vi "Package Information Pre Build Action.vi"(10 "Variant":variant) -> (0 "error out":errorcluster)   [LabVIEW 2017, in "CL_G3_VIComponentBuilder.lvlib"]
uses:
  CL_G3_VIComponentBuilder.lvlib
  <vilib>/LVH/i3 JSON/JSON Parsing/Get Object Parameter Files/Get Object Parameter - Object.vi
  <vilib>/LVH/i3 JSON/JSON Parsing/Get Object Parameter Files/Get Object Parameter - Boolean.vi
  VIPM Utilities/CL_G3_VIPMUtilities.lvlib
  <vilib>/LVH/i3 JSON/i3-json.lvlib
panel:
  out "String":string
  out "Total":i32
  out "Progress":i32(slide) scale=-1.0..85.0
  # "Adding Package details to VI description"
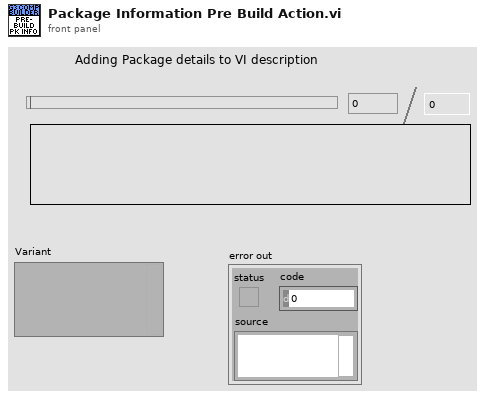
[diagram p1: front panel]
types:
  T1 = enum32{"Invalid", "Standard", "Closed", "Hidden", "Minimized", "Maximized"}
  T2 = cluster{"Error State":errorcluster, "Processed Documentation":string, "Build Spec Path":path, "VIs In Package":path[], "Product Name":string, "Package Version":string, "Package Name":string, "Current File to process":path, "vi reference being processed":refnum<vi>, "Opened References":refnum<vi>[], "Build Options i3JSON Tree":variant}
  T3 = cluster{"Beginning of Tag Position":i32, "End of Tag Position":i32}[]
  T4 = cluster{"Beginning of Tag Position":i32, "End of Tag Position":i32}
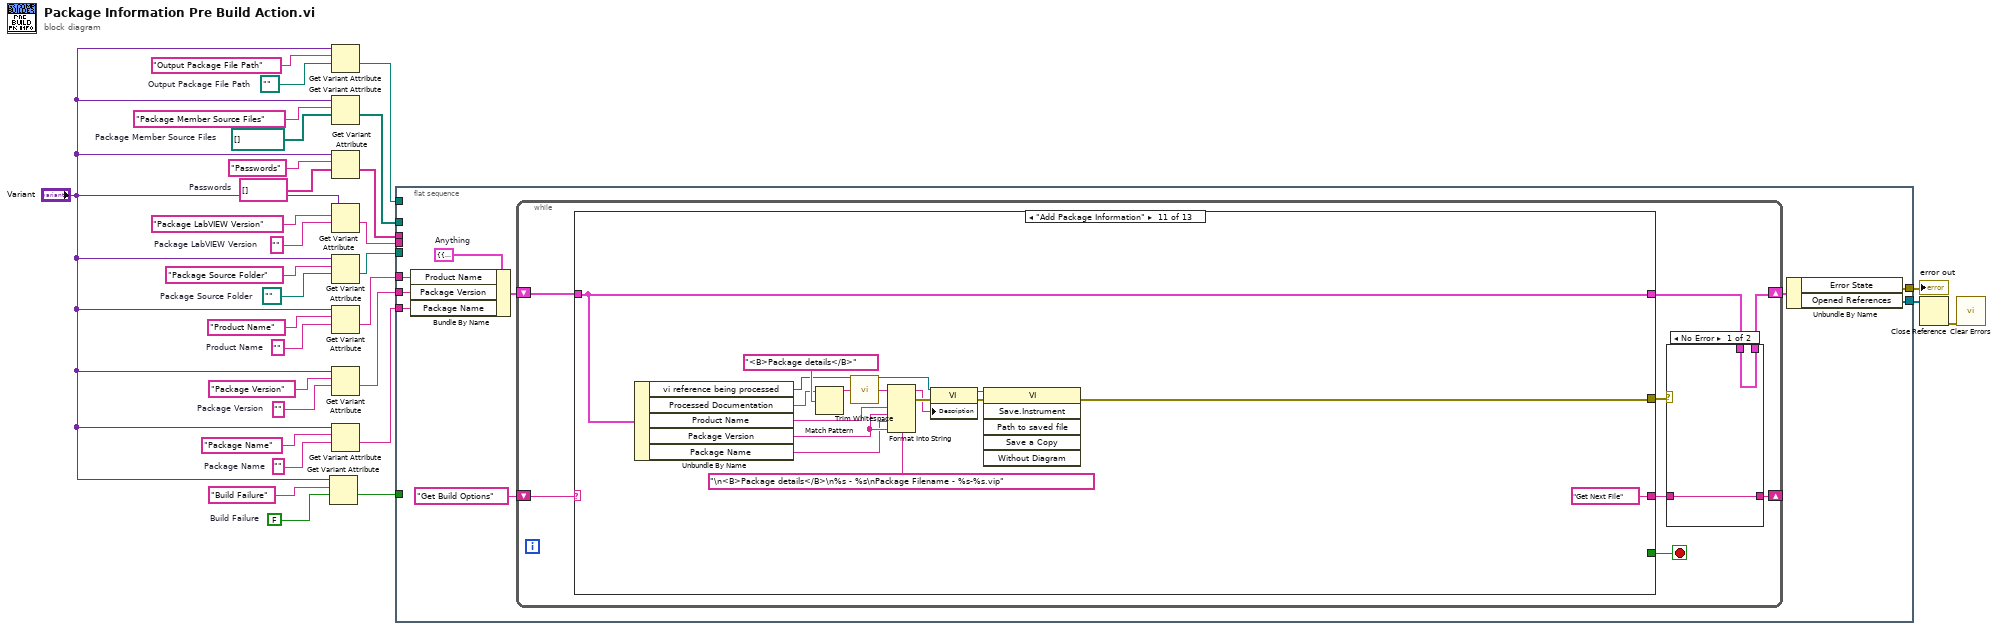
[diagram p0: block diagram]
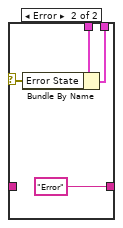
[diagram p2: hidden frame]
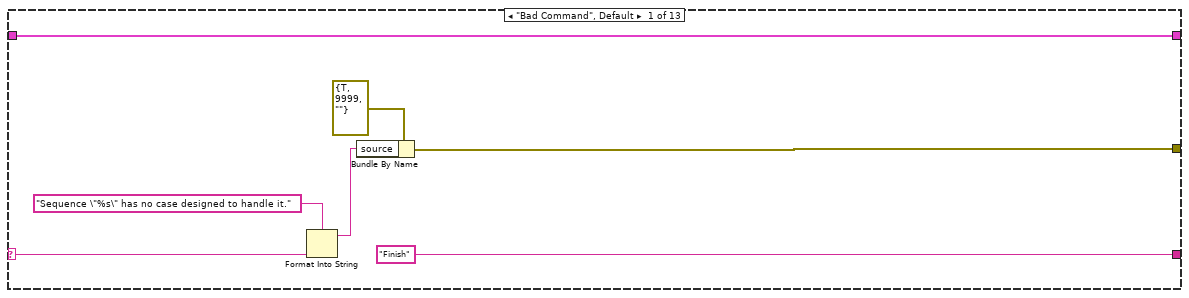
[diagram p3: hidden frame]
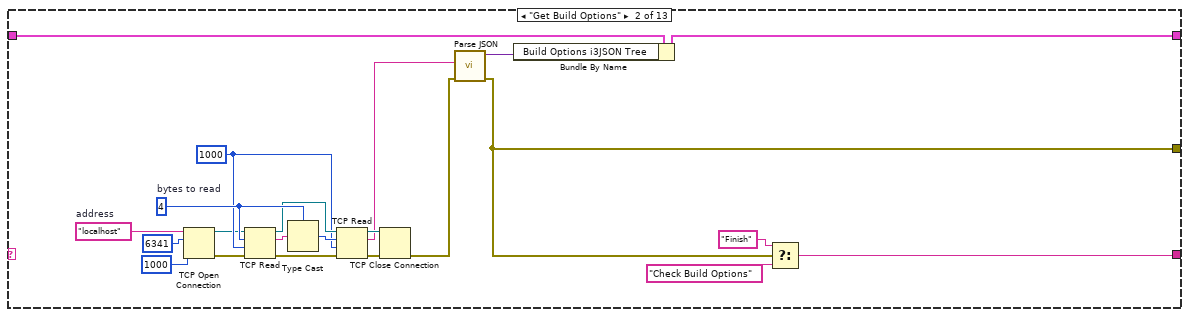
[diagram p4: hidden frame]
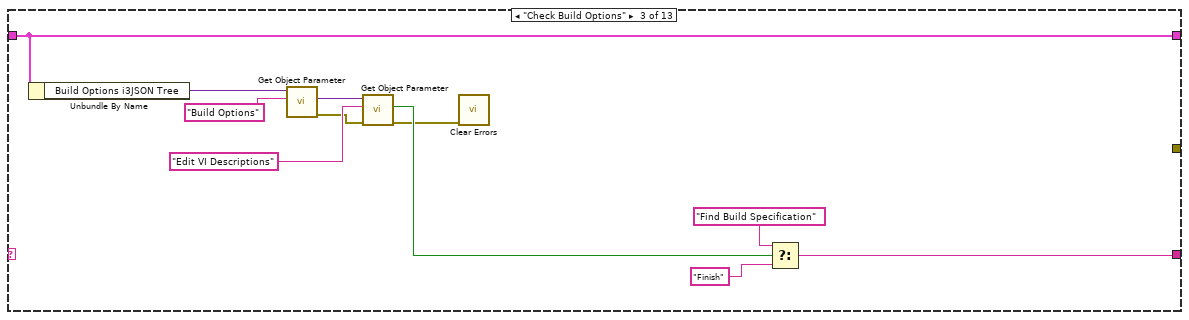
[diagram p5: hidden frame]
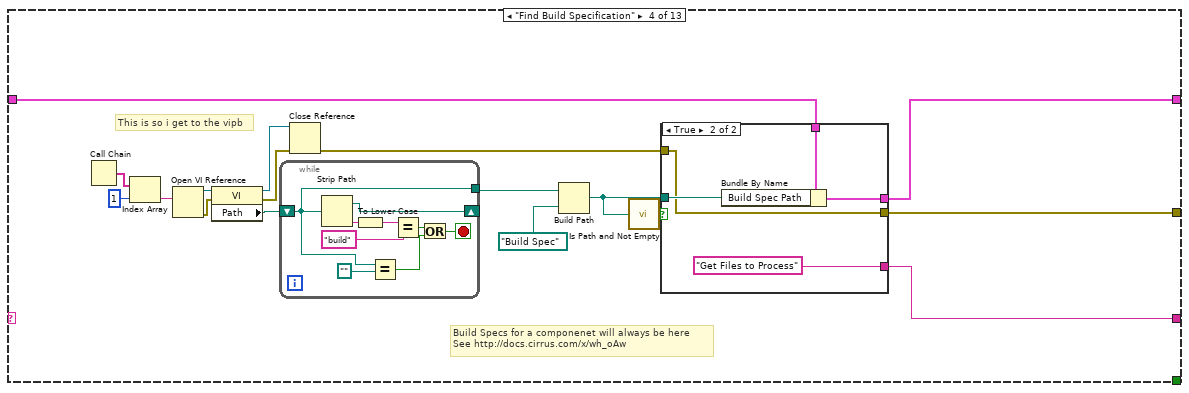
[diagram p6: hidden frame]
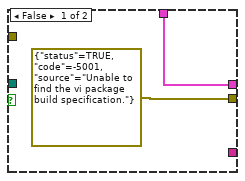
[diagram p7: hidden frame]
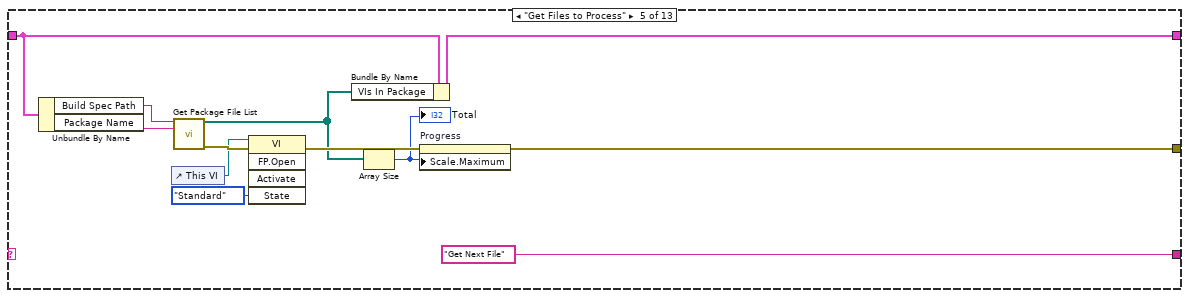
[diagram p8: hidden frame]
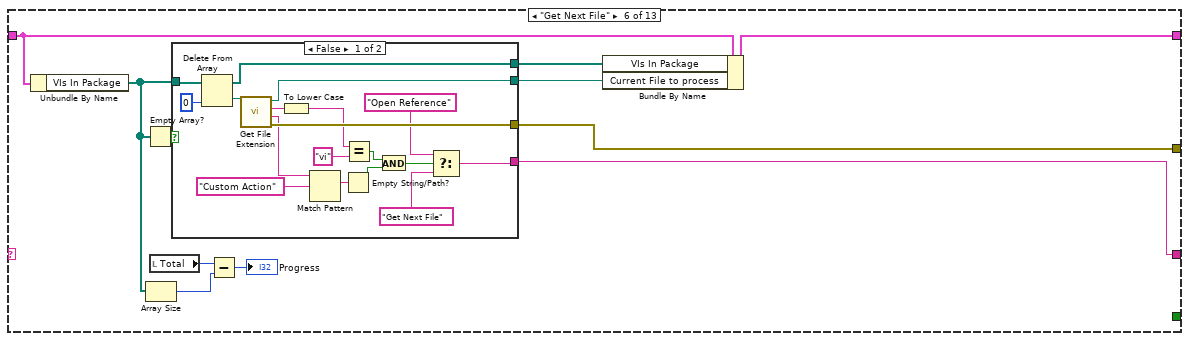
[diagram p9: hidden frame]
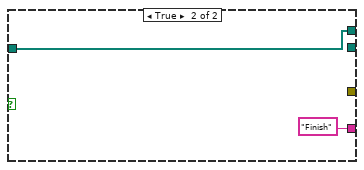
[diagram p10: hidden frame]
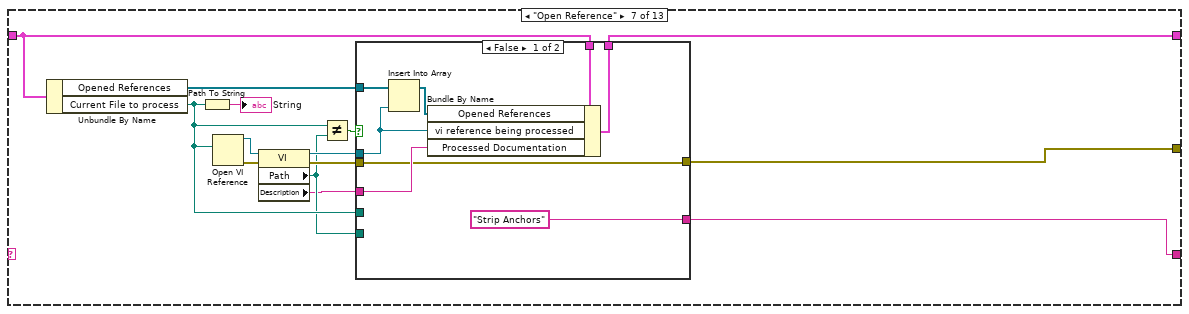
[diagram p11: hidden frame]
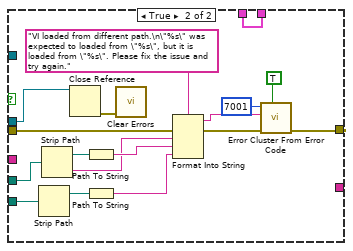
[diagram p12: hidden frame]
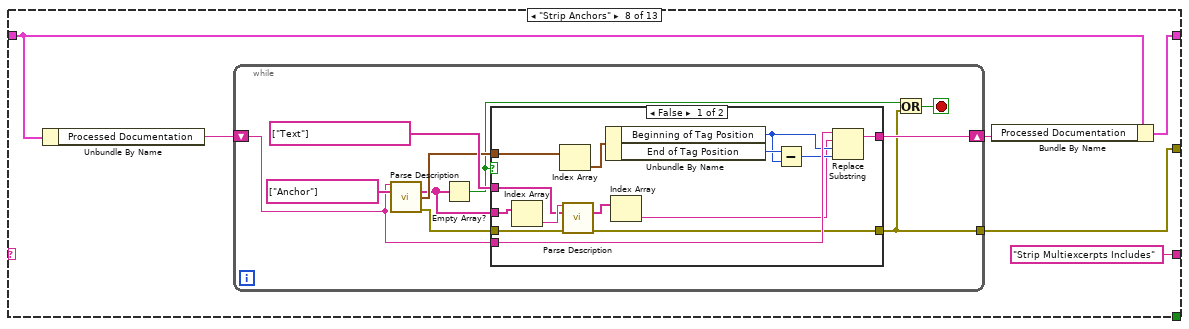
[diagram p13: hidden frame]
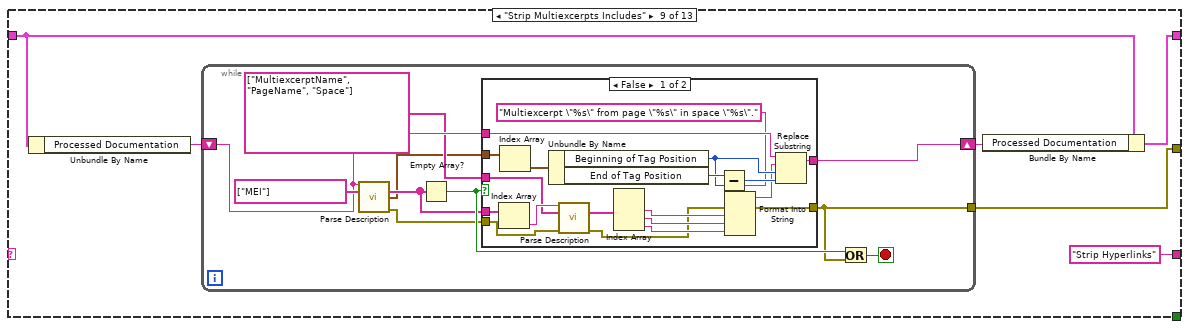
[diagram p15: hidden frame]
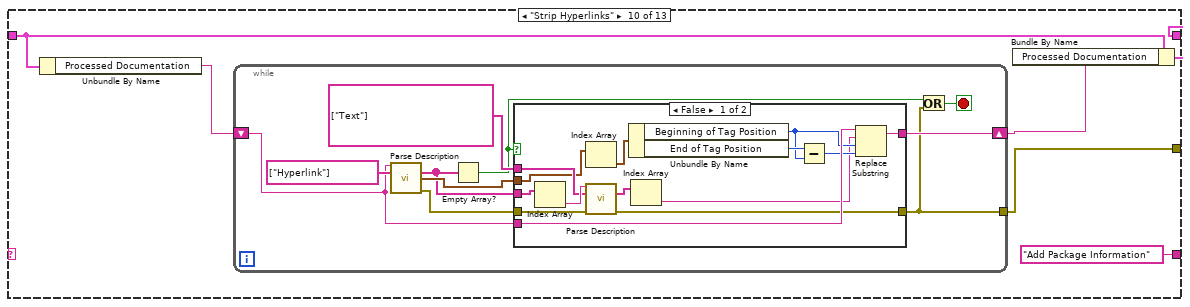
[diagram p17: hidden frame]
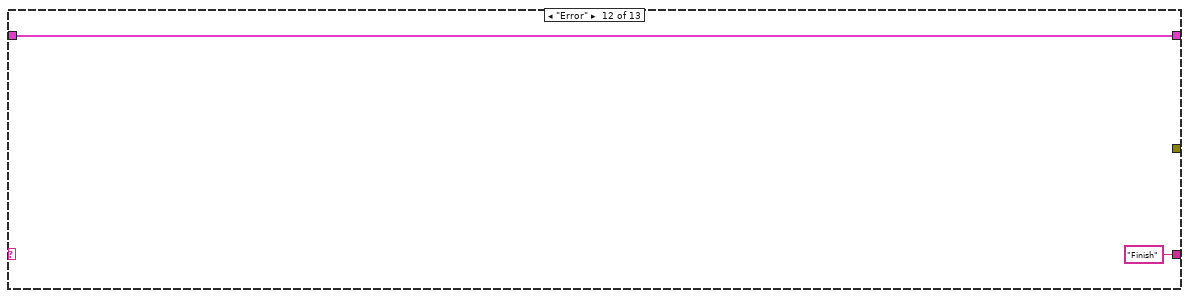
[diagram p19: hidden frame]
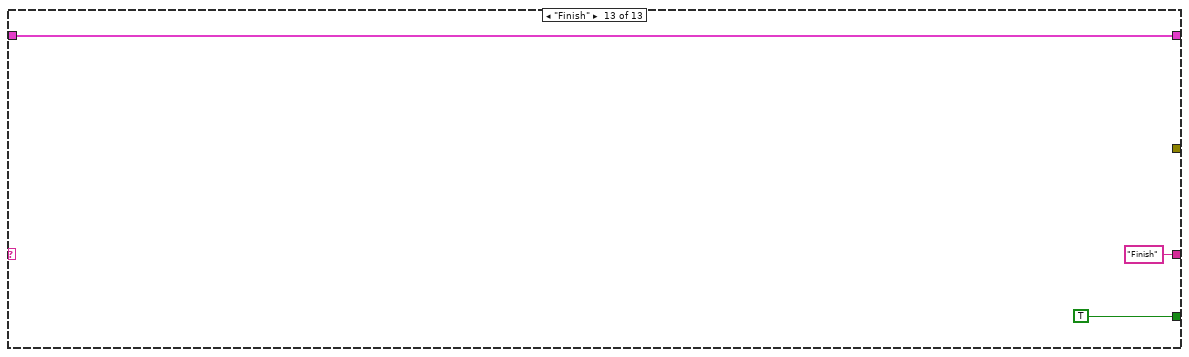
[diagram p20: hidden frame]
diagram:
  w14 = FALSE  # Build Failure
  w16 = path ""  # Package Source Folder
  w17 = ""  # Package Name
  w20 = ""  # Package LabVIEW Version
  w22 = ""  # Package Version
  w24 = ""  # Product Name
  w26 = string[] []  # Passwords
  w28 = path[] []  # Package Member Source Files
  w30 = path ""  # Output Package File Path
  n1 = Get Variant Attribute(Variant="Variant", name="Build Failure", default value (empty Variant)=w14) -> (value=w1:bool)  [unwired: 1 in, 3 out]
  n2 = Get Variant Attribute(Variant="Variant", name="Output Package File Path", default value (empty Variant)=w30) -> (value=w6:path)  [unwired: 1 in, 3 out]
  n3 = Get Variant Attribute(Variant="Variant", name="Package Member Source Files", default value (empty Variant)=w28) -> (value=w5:path[])  [unwired: 1 in, 3 out]
  n4 = Get Variant Attribute(Variant="Variant", name="Passwords", default value (empty Variant)=w26) -> (value=w4:string[])  [unwired: 1 in, 3 out]
  n5 = Get Variant Attribute(Variant="Variant", name="Package LabVIEW Version", default value (empty Variant)=w20) -> (value=w3:string)  [unwired: 1 in, 3 out]
  n6 = Get Variant Attribute(Variant="Variant", name="Package Source Folder", default value (empty Variant)=w16) -> (value=w2:path)  [unwired: 1 in, 3 out]
  n7 = Get Variant Attribute(Variant="Variant", name="Product Name", default value (empty Variant)=w24) -> (value=w12:string)  [unwired: 1 in, 3 out]
  n8 = Get Variant Attribute(Variant="Variant", name="Package Version", default value (empty Variant)=w22) -> (value=w11:string)  [unwired: 1 in, 3 out]
  n9 = Get Variant Attribute(Variant="Variant", name="Package Name", default value (empty Variant)=w17) -> (value=w10:string)  [unwired: 1 in, 3 out]
  n10 = flat-sequence {
    tunnel: w12 -> [w38]
    tunnel: w11 -> [w37]
    tunnel: w10 -> [w36]
    tunnel: [w34] -> w9
    tunnel: [w33] -> w8
    tunnel: w6 -> [_]
    tunnel: w5 -> [_]
    tunnel: w4 -> [_]
    tunnel: w3 -> [_]
    tunnel: w2 -> [_]
    tunnel: w1 -> [_]
    frame #0 {
      w32 = T2 {"Error State"={"status"=FALSE, "code"=0, "source"=""}, "Processed Documentation"="", "Build Spec Path"=path "", "VIs In Package"=[], "Product Name"="", "Package Version"="", "Package Name"="", "Current File to process"=path "", "vi reference being processed"=refnum, "Opened References"=[], "Build Options i3JSON Tree"=variant}  # Anything
      n11 = Bundle By Name(cluster=w32, "Product Name"=w38, "Package Version"=w37, "Package Name"=w36) -> (w40:T2)
      n12 = while {
        shift-right: [w43] -> w39
        shift-left: w40 -> [w48]
        shift-right: [w42] -> _
        shift-left: "Get Build Options" -> [w47]
        stop <- w41 stop-if-true
        n13 = case shown="\"Add Package Information\"" w47 {
          selector: w47 -> [w58 _ _ _ _ _ _ _ _ _ _ _ _]
          tunnel: w48 -> [w61 w83 w91 w100 w131 w150 w175 w215 w246 w283 w315 w326 w329]
          tunnel: [w61 w67 w91 w101 w135 w149 w174 w213 w244 w281 w315 w326 w329] -> w44
          tunnel: ["Finish" ("Accessors:Name") w82 w92 w99 "Get Next File" w145 w173 "Strip Multiexcerpts Includes" ("y") "Strip Hyperlinks" ("y") "Add Package Information" ("y") "Get Next File" ("y") "Finish" "Finish"] -> w46
          tunnel: [w56 w64 _ w97 w133 w147 w178 w211 w241 w278 w310 _ _] -> w45
          tunnel: [_ _ _ _ _ _ _ _ _ _ _ _ TRUE] -> w41
          frame "Bad Command", Default {
            n14 = Format Into String(format string="Sequence \"%s\" has no case designed to handle it.", w58) -> (resulting string=w57:string)  [unwired: 2 in, 1 out]
            n15 = Bundle By Name(cluster=errorcluster {"status"=TRUE, "code"=9999, "source"=""} ("error out"), "source"=w57) -> (w56:errorcluster)
          }
          frame "Get Build Options" {
            w74 = 1000 ("timeout ms (25000)")
            w78 = 4  # bytes to read
            w81 = "localhost"  # address
            n16 = TCP Open Connection(address=w81, remote port or service name=u16 6341, timeout ms (60000)=1000) -> (connection ID=w73:refnum<k5>, error out=w72:errorcluster)  [unwired: 2 in]
            n17 = TCP Read(connection ID=w73, bytes to read=w78, error in (no error)=w72, 9:w74) -> (connection ID out=w77:refnum<k5>, data out=w79:string, error out=w76:errorcluster)  [unwired: 1 in]
            n18 = Type Cast(type=w78, x=w79) -> (*(type *) &x=w75:i32)
            n19 = TCP Read(connection ID=w77, bytes to read=w75, error in (no error)=w76, 9:w74) -> (connection ID out=w71:refnum<k5>, data out=w69:string, error out=w70:errorcluster)  [unwired: 1 in]
            n20 = TCP Close Connection(connection ID=w71, error in (no error)=w70) -> (error out=w65:errorcluster)  [unwired: 1 in, 1 out]
            n21 = call <vilib>:"Parse JSON.vi"("error in (no error)"=w65, "JSON String"=w69) -> ("error out"=w64:errorcluster, "JSON Tree"=w66:variant)  [unwired: 6 in, 2 out]
            n22 = Bundle By Name(cluster=w83, "Build Options i3JSON Tree"=w66) -> (w67:T2)
            n23 = Select(t="Finish", s=w64, f="Check Build Options") -> (s? t:f=w82:string)
          }
          frame "Check Build Options" {
            n24 = Unbundle By Name(w91) -> ("Build Options i3JSON Tree"=w90:variant)
            n25 = call-poly <vilib>:"Get Object Parameter.vi"("Parameter Name"="Build Options", "JSON Tree In (JSON Object)"=w90) -> ("error out"=w85:errorcluster, "JSON Object"=w89:variant)  [unwired: 6 in, 2 out]
            n26 = call-poly <vilib>:"Get Object Parameter.vi"("error in (no error)"=w85, "Parameter Name"="Edit VI Descriptions" ("Option Name"), "JSON Tree In (JSON Object)"=w89) -> ("error out"=w84:errorcluster, "Boolean Value"=w86:bool)  [unwired: 5 in, 2 out]
            n27 = call <vilib>:"Clear Errors.vi"("error in (no error)"=w84) -> ()  [unwired: 5 in, 2 out]
            n28 = Select(t="Find Build Specification", s=w86, f="Finish") -> (s? t:f=w92:string)
          }
          frame "Find Build Specification" {
            # "This is so i get to the vipb"
            # "Build Specs for a componenet will always be here\nSee http://docs.cirrus.com/x/wh_oAw"
            n29 = Call Chain() -> (call chain=w109:string[])
            n30 = Index Array(array=w109, index=1) -> (element=w105:string)
            n31 = Open VI Reference(vi path=w105) -> (vi reference=w106:refnum<vi>, error out=w98:errorcluster)  [unwired: 5 in]
            n32 = property class="VI"(reference=w106, error in=w98) -> (reference out=w107:refnum<vi>, error out=w96:errorcluster, "Path"=w108:path)
            n33 = while {
              shift-right: [w122] -> _
              shift-left: w108 -> [w120]
              tunnel: [w120] -> w111
              stop <- w127 stop-if-true
              n34 = Strip Path(path=w120) -> (stripped path=w122:path, name=w126:string)
              n35 = To Lower Case(string=w126) -> (all lower case string=w125:string)
              n36 = Equal?(x=w120, y=path "") -> (x = y?=w119:bool)
              n37 = Equal?(x=w125, y="build") -> (x = y?=w123:bool)
              n38 = Or(x=w123, y=w119) -> (x .or. y?=w127:bool)
            }
            n39 = Close Reference(reference=w107, error in (no error)=w96) -> (error out=w95:errorcluster)
            n40 = Build Path(base path=w111, name or relative path=path "Build Spec" ("VIPB Folder")) -> (appended path=w102:path)
            n41 = call <vilib>:"Is Path and Not Empty.vi"("path"=w102) -> ("Is Path and Not Empty?"=w103:bool)  [unwired: 4 in]
            n42 = case shown="True" w103 {
              tunnel: [_ "Get Files to Process"] -> w99
              tunnel: w102 -> [_ w117]
              tunnel: w100 -> [w112 w116]
              tunnel: [w112 w115] -> w101
              tunnel: [errorcluster {"status"=TRUE, "code"=-5001, "source"="Unable to find the vi package build specification."} ("Error State") w114] -> w97
              tunnel: w95 -> [_ w114]
              frame False {
              }
              frame True {
                n43 = Bundle By Name(cluster=w116, "Build Spec Path"=w117) -> (w115:T2)
              }
            }
          }
          frame "Get Files to Process" {
            n44 = Unbundle By Name(w131) -> ("Build Spec Path"=w130:path, "Package Name"=w129:string)
            n45 = control-ref of="This VI"() -> (w136:refnum<vi>)
            n46 = call "Get Package File List.vi"("VIPB Folder"=w130, "Package Name"=w129) -> ("Included Files"=w134:path[], "error out"=w139:errorcluster)  [unwired: 12 in]
            n47 = invoke class="VI" method="FP.Open"(reference=w136, error in=w139, "State"=T1."Standard") -> (error out=w138:errorcluster)  [unwired: 2 in, 4 out]
            n48 = Bundle By Name(cluster=w131, "VIs In Package"=w134) -> (w135:T2)
            n49 = Array Size(array=w134) -> (size(s)=w132:i32)
            "Total" <- w132
            n50 = property on="Progress" class="Slide (strict)"(error in=w138, "Scale.Maximum"=w132) -> (error out=w133:errorcluster)  [unwired: 1 in, 1 out]
          }
          frame "Get Next File" {
            n51 = Unbundle By Name(w150) -> ("VIs In Package"=w143:path[])
            n52 = Empty Array?(array=w143) -> (empty?=w146:bool)
            n53 = Array Size(array=w143) -> (size(s)=w142:i32)
            n54 = local read "Total"() -> (w141:i32)
            n55 = case shown="False" w146 {
              tunnel: [w165 _] -> w148
              tunnel: [w164 _] -> w147
              tunnel: w143 -> [w157 w169]
              tunnel: [w153 "Finish" ("y")] -> w145
              tunnel: [w152 w169] -> w144
              frame False {
                n56 = Delete From Array(array=w157, index=0) -> (deleted portion=w166:path, array with subset deleted=w152:path[])  [unwired: 1 in]
                n57 = call <vilib>:"Get File Extension.vi"("file"=w166) -> ("error out"=w164:errorcluster, "filename without extension"=w163:string, "lowercase file extension"=w162:string, "dup file"=w165:path)  [unwired: 6 in, 1 out]
                n58 = To Lower Case(string=w162) -> (all lower case string=w160:string)
                n59 = Match Pattern(string=w163, regular expression="Custom Action") -> (match substring=w168:string)  [unwired: 1 in, 3 out]
                n60 = Empty String/Path?(string/path=w168) -> (empty?=w158:bool)
                n61 = Equal?(x=w160, y="vi") -> (x = y?=w159:bool)
                n62 = And(x=w159, y=w158) -> (x .and. y?=w156:bool)
                n63 = Select(t="Open Reference" ("y"), s=w156, f="Get Next File" ("y")) -> (s? t:f=w153:string)
              }
              frame True {
              }
            }
            n64 = Subtract(x=w141, y=w142) -> (x-y=→"Progress":i32)
            n65 = Bundle By Name(cluster=w150, "VIs In Package"=w144, "Current File to process"=w148) -> (w149:T2)
          }
          frame "Open Reference" {
            n66 = Unbundle By Name(w175) -> ("Opened References"=w171:refnum<vi>[], "Current File to process"=w177:path)
            n67 = Path To String(path=w177) -> (string=→"String":string)
            n68 = Open VI Reference(vi path=w177) -> (vi reference=w184:refnum<vi>, error out=w183:errorcluster)  [unwired: 5 in]
            n69 = property class="VI"(reference=w184, error in=w183) -> (reference out=w180:refnum<vi>, error out=w179:errorcluster, "Path"=w176:path, "Description"=w172:string)
            n70 = Not Equal?(x=w177, y=w176) -> (x != y?=w181:bool)
            n71 = case shown="False" w181 {
              tunnel: w180 -> [w187 w195]
              tunnel: w179 -> [w185 w199]
              tunnel: [w185 w198] -> w178
              tunnel: w177 -> [_ w197]
              tunnel: w176 -> [_ w196]
              tunnel: w175 -> [w192 w193]
              tunnel: [w191 w193] -> w174
              tunnel: ["Strip Anchors" _] -> w173
              tunnel: w172 -> [w189 _]
              tunnel: w171 -> [w188 _]
              frame False {
                n72 = Insert Into Array(array=w188, new element=w187) -> (w186:refnum<vi>[])  [unwired: 1 in]
                n73 = Bundle By Name(cluster=w192, "Opened References"=w186, "vi reference being processed"=w187, "Processed Documentation"=w189) -> (w191:T2)
              }
              frame True {
                n74 = Strip Path(path=w196) -> (stripped path=w205:path)  [unwired: 1 out]
                n75 = Strip Path(path=w197) -> (stripped path=w203:path, name=w202:string)
                n76 = Close Reference(reference=w195) -> (error out=w194:errorcluster)  [unwired: 1 in]
                n77 = Path To String(path=w203) -> (string=w204:string)
                n78 = Path To String(path=w205) -> (string=w206:string)
                n79 = call <vilib>:"Clear Errors.vi"("error in (no error)"=w194) -> ()  [unwired: 5 in, 2 out]
                n80 = Format Into String(format string="VI loaded from different path.\n\"%s\" was expected to loaded from \"%s\", but it is loaded from \"%s\". Please fix the issue and try again.", error in=w199, w202, w204, w206) -> (resulting string=w207:string, error out=w200:errorcluster)  [unwired: 1 in]
                n81 = call <vilib>:"Error Cluster From Error Code.vi"("show call chain? (False)"=TRUE, "error in (no error)"=w200, "error message (\"\")"=w207, "error code (0)"=7001) -> ("error out"=w198:errorcluster)  [unwired: 5 in]
              }
            }
          }
          frame "Strip Anchors" {
            n82 = Unbundle By Name(w215) -> ("Processed Documentation"=w214:string)
            n83 = while {
              shift-right: [w221] -> w212
              shift-left: w214 -> [w222]
              tunnel: [w218] -> w211
              stop <- w216 stop-if-true
              n84 = call "Parse Description.vi"("Description"=w222, "XML Values to Parse"=string[] ["Anchor"]) -> ("XML Values"=w219:string[], "String Bounds of Matches"=w223:T3, "error out"=w220:errorcluster)  [unwired: 10 in, 1 out]
              n85 = Empty Array?(array=w219) -> (empty?=w217:bool)
              n86 = case shown="False" w217 {
                tunnel: w219 -> [w239 _]
                tunnel: w220 -> [w236 _]
                tunnel: string[] ["Text"] ("XML Values to Parse") -> [w235 _]
                tunnel: w223 -> [w234 _]
                tunnel: w222 -> [w233 w240]
                tunnel: [w232 w240] -> w221
                tunnel: [w226 _] -> w218
                frame False {
                  n87 = Index Array(array=w239) -> (element=w238:string)  [unwired: 1 in]
                  n88 = Index Array(array=w234) -> (element=w231:T4)  [unwired: 1 in]
                  n89 = call "Parse Description.vi"("Description"=w238, "XML Values to Parse"=w235, "error in (no error) 2"=w236) -> ("XML Values"=w237:string[], "error out"=w226:errorcluster)  [unwired: 9 in, 2 out]
                  n90 = Unbundle By Name(w231) -> ("Beginning of Tag Position"=w229:i32, "End of Tag Position"=w230:i32)
                  n91 = Index Array(array=w237) -> (element=w227:string)  [unwired: 1 in]
                  n92 = Subtract(x=w230, y=w229) -> (x-y=w228:i32)
                  n93 = Replace Substring(2:w228, 3:w229, 4:w227, 5:w233) -> (1:w232:string)  [unwired: 1 out]
                }
                frame True {
                }
              }
              n94 = Or(x=w217, y=w218) -> (x .or. y?=w216:bool)
            }
            n95 = Bundle By Name(cluster=w215, "Processed Documentation"=w212) -> (w213:T2)
          }
          frame "Strip Multiexcerpts Includes" {
            n96 = Unbundle By Name(w246) -> ("Processed Documentation"=w245:string)
            n97 = while {
              shift-right: [w254] -> w243
              shift-left: w245 -> [w255]
              tunnel: [w247] -> w241
              stop <- w252 stop-if-true
              n98 = call "Parse Description.vi"("Description"=w255, "XML Values to Parse"=string[] ["MEI"]) -> ("XML Values"=w251:string[], "String Bounds of Matches"=w249:T3, "error out"=w248:errorcluster)  [unwired: 10 in, 1 out]
              n99 = Empty Array?(array=w251) -> (empty?=w253:bool)
              n100 = case shown="False" w253 {
                tunnel: w249 -> [w275 _]
                tunnel: w255 -> [w274 w277]
                tunnel: [w273 w277] -> w254
                tunnel: w251 -> [w268 _]
                tunnel: string[] ["MultiexcerptName", "PageName", "Space"] ("XML Values to Parse") -> [w266 _]
                tunnel: [w258 w276] -> w247
                tunnel: w248 -> [w257 w276]
                frame False {
                  n101 = Index Array(array=w268) -> (element=w267:string)  [unwired: 1 in]
                  n102 = Index Array(array=w275) -> (element=w272:T4)  [unwired: 1 in]
                  n103 = Unbundle By Name(w272) -> ("Beginning of Tag Position"=w270:i32, "End of Tag Position"=w271:i32)
                  n104 = call "Parse Description.vi"("Description"=w267, "XML Values to Parse"=w266, "error in (no error) 2"=w257) -> ("XML Values"=w265:string[], "error out"=w259:errorcluster)  [unwired: 9 in, 2 out]
                  n105 = Index Array(array=w265) -> (element #1=w264:string, element #2=w263:string, element #3=w262:string)  [unwired: 3 in]
                  n106 = Subtract(x=w271, y=w270) -> (x-y=w269:i32)
                  n107 = Format Into String(format string="Multiexcerpt \"%s\" from page \"%s\" in space \"%s\".", error in=w259, w264, w263, w262) -> (resulting string=w260:string, error out=w258:errorcluster)  [unwired: 1 in]
                  n108 = Replace Substring(2:w269, 3:w270, 4:w260, 5:w274) -> (1:w273:string)  [unwired: 1 out]
                }
                frame True {
                }
              }
              n109 = Or(x=w253, y=w247) -> (x .or. y?=w252:bool)
            }
            n110 = Bundle By Name(cluster=w246, "Processed Documentation"=w243) -> (w244:T2)
          }
          frame "Strip Hyperlinks" {
            n111 = Unbundle By Name(w283) -> ("Processed Documentation"=w282:string)
            n112 = while {
              shift-right: [w289] -> w280
              shift-left: w282 -> [w290]
              tunnel: [w286] -> w278
              stop <- w285 stop-if-true
              n113 = call "Parse Description.vi"("Description"=w290, "XML Values to Parse"=string[] ["Hyperlink"]) -> ("XML Values"=w287:string[], "String Bounds of Matches"=w291:T3, "error out"=w288:errorcluster)  [unwired: 10 in, 1 out]
              n114 = Empty Array?(array=w287) -> (empty?=w284:bool)
              n115 = case shown="False" w284 {
                tunnel: w287 -> [w307 _]
                tunnel: w288 -> [w304 _]
                tunnel: string[] ["Text"] ("XML Values to Parse") -> [w303 _]
                tunnel: w291 -> [w302 _]
                tunnel: w290 -> [w301 w308]
                tunnel: [w300 w308] -> w289
                tunnel: [w294 _] -> w286
                frame False {
                  n116 = Index Array(array=w307) -> (element=w306:string)  [unwired: 1 in]
                  n117 = Index Array(array=w302) -> (element=w299:T4)  [unwired: 1 in]
                  n118 = call "Parse Description.vi"("Description"=w306, "XML Values to Parse"=w303, "error in (no error) 2"=w304) -> ("XML Values"=w305:string[], "error out"=w294:errorcluster)  [unwired: 9 in, 2 out]
                  n119 = Unbundle By Name(w299) -> ("Beginning of Tag Position"=w297:i32, "End of Tag Position"=w298:i32)
                  n120 = Index Array(array=w305) -> (element=w295:string)  [unwired: 1 in]
                  n121 = Subtract(x=w298, y=w297) -> (x-y=w296:i32)
                  n122 = Replace Substring(2:w296, 3:w297, 4:w295, 5:w301) -> (1:w300:string)  [unwired: 1 out]
                }
                frame True {
                }
              }
              n123 = Or(x=w284, y=w286) -> (x .or. y?=w285:bool)
            }
            n124 = Bundle By Name(cluster=w283, "Processed Documentation"=w280) -> (w281:T2)
          }
          frame "Add Package Information" {
            n125 = Unbundle By Name(w315) -> ("vi reference being processed"=w309:refnum<vi>, "Processed Documentation"=w314:string, "Product Name"=w313:string, "Package Version"=w312:string, "Package Name"=w311:string)
            n126 = Match Pattern(string=w314, regular expression="<B>Package details</B>") -> (before substring=w318:string)  [unwired: 1 in, 3 out]
            n127 = call <vilib>:"Trim Whitespace.vi"("string"=w318) -> ("trimmed string"=w317:string)  [unwired: 1 in]
            n128 = Format Into String(format string="\n<B>Package details</B>\n%s - %s\nPackage Filename - %s-%s.vip", initial string=w317, w313, w312, w311, w312) -> (resulting string=w321:string, error out=w322:errorcluster)  [unwired: 1 in]
            n129 = property class="VI"(reference=w309, error in=w322, "Description"=w321) -> (reference out=w320:refnum<vi>, error out=w323:errorcluster)
            n130 = invoke class="VI" method="Save.Instrument"(reference=w320, error in=w323) -> (error out=w310:errorcluster)  [unwired: 4 in, 5 out]
          }
          frame "Error" {
          }
          frame "Finish" {
          }
        }
        n131 = case shown="No Error" w45 {
          selector: w45 -> [_ w54]
          tunnel: w46 -> [w50 _]
          tunnel: [w50 "Error"] -> w42
          tunnel: w44 -> [w49 w53]
          tunnel: [w49 w52] -> w43
          frame No Error {
          }
          frame Error {
            n132 = Bundle By Name(cluster=w53, "Error State"=w54) -> (w52:T2)
          }
        }
      }
      n133 = Unbundle By Name(w39) -> ("Error State"=w33:errorcluster, "Opened References"=w34:refnum<vi>[])
    }
  }
  n134 = Close Reference(reference=w9) -> (error out=w7:errorcluster)  [unwired: 1 in]
  n135 = call <vilib>:"Clear Errors.vi"("error in (no error)"=w7) -> ()  [unwired: 5 in, 2 out]
  "error out" <- w8
